vi "QSM_INIT_UpdateUI.vi"(7 "user event in":refnum<user-event>, 8 "error in":errorcluster, 9 "FP References":T1, 11 "Queue References":T3) -> (0 "error out":errorcluster, 3 "QSM_ShiftRegister":T2)   [LabVIEW 2014, in "GUIUpdateQSM.lvlib"]
doc: "DISPLAY 'DISP' Queued State Machine Shift Register Data:\n\nThe data type for the main shift register in the subsequent queued state machine is defined in large clusters within this VI."
uses:
  GUIUpdateQSM.lvlib
  QueueMaintenance/TypeDef/QSMRef_ALL.ctl
  Controls/QSM_Reference.ctl
  Controls/QSM_DataType.ctl
  Controls/QSM_RunStates.ctl
  Queue_TEST/Controls/QSM_Reference.ctl
  Queue_TEST/Controls/QSM_DataType.ctl
  Queue_TEST/Controls/QSM_RunStates.ctl
  Controls/QSM_ShiftRegister.ctl
  Controls/TypeDef_FrontPanelReferences.ctl
  QueueMaintenance/QueueMaintenance.lvlib
  Queue_TEST/TestQSM.lvlib
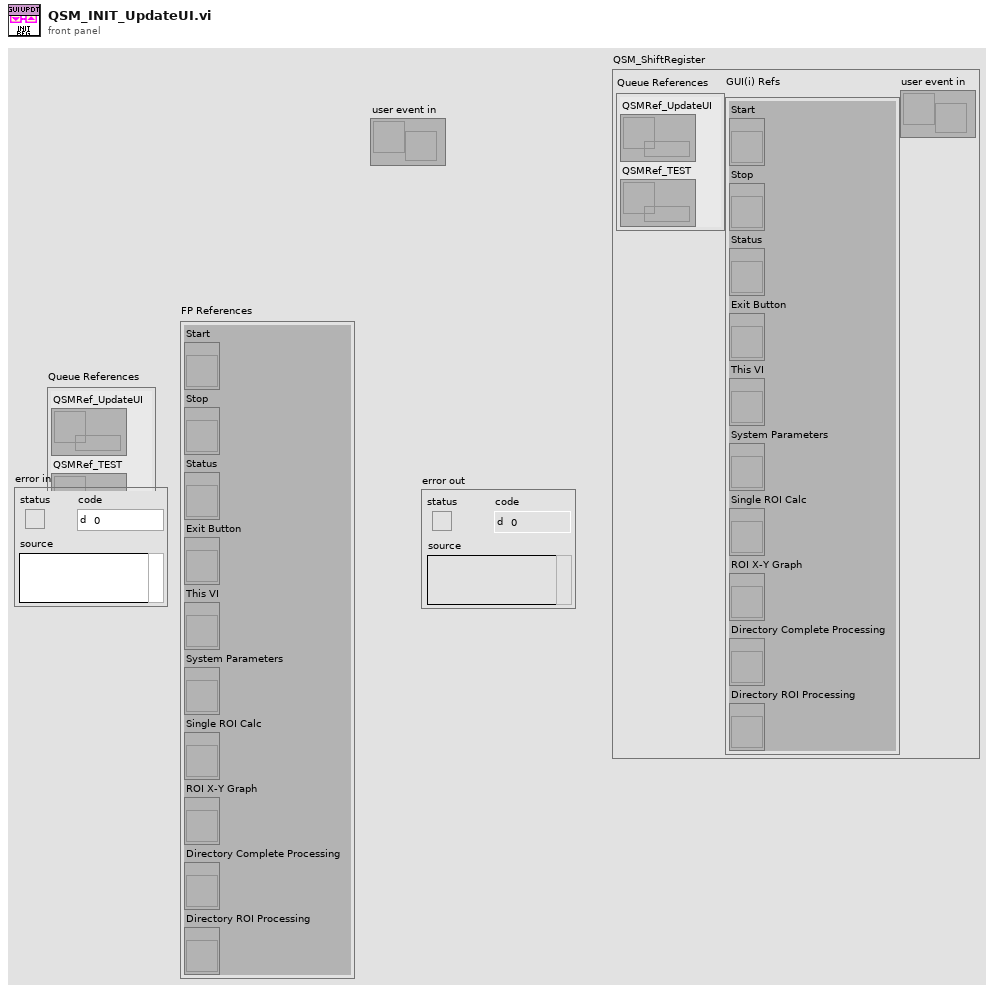
[diagram p1: front panel]
types:
  T1 = typedef "GUIUpdateQSM.lvlib/TypeDef_FrontPanelReferences.ctl" = cluster{"Start":refnum<vi>, "Stop":refnum<vi>, "Status":refnum<vi>, "Exit Button":refnum<vi>, "This VI":refnum<vi>, "System Parameters":refnum<vi>, "Single ROI Calc":refnum<vi>, "ROI X-Y Graph":refnum<vi>, "Directory Complete Processing":refnum<vi>, "Directory ROI Processing":refnum<vi>}
  T2 = typedef "GUIUpdateQSM.lvlib/QSM_ShiftRegister.ctl" = cluster{"Queue References":T3, "GUI(i) Refs":T1, "user event in":refnum<user-event>}
  T3 = typedef "QueueMaintenance.lvlib/QSMRef_ALL.ctl" = cluster{"QSMRef_UpdateUI":T4, "QSMRef_TEST":T5}
  T4 = typedef "GUIUpdateQSM.lvlib/QSM_Reference.ctl" = refnum<queue>
  T5 = typedef "TestQSM.lvlib/QSM_Reference.ctl" = refnum<queue>
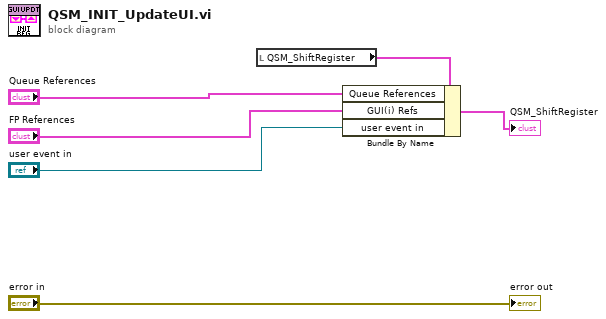
[diagram p0: block diagram]
diagram:
  n1 = local read "QSM_ShiftRegister"() -> (w3:T2)
  n2 = Bundle By Name(cluster=w3, "Queue References"="Queue References", "GUI(i) Refs"="FP References", "user event in"="user event in") -> (→"QSM_ShiftRegister":T2)
  "error out" <- "error in"
